vi "COMI DO Put One.vi"(9 "status":i32, 10 "ch":i32, 11 "hDevice":u32) -> (2 "function return":i32, 3 "hDevice out":u32)   [LabVIEW 2017, in "Comidll.lvlib"]
doc: "int (COMI_DO_PutOne) (HANDLE hDevice, int ch, int status);"
uses:
  <userlib>/Comidll/Comidll.lvlib
  <userlib>/Comidll/Comidll.dll
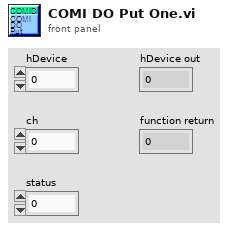
[diagram p1: front panel]
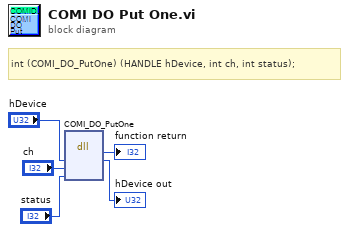
[diagram p0: block diagram]
diagram:
  # "int\t(COMI_DO_PutOne) (HANDLE hDevice, int ch, int status);"
  n1 = dll-call lib="C:/Program Files/National Instruments/LabVIEW 2017/user.lib/Comidll/Comidll.*" fn="COMI_DO_PutOne"("hDevice"="hDevice", "ch"="ch", "status"="status") -> (→"function return":i32, "hDevice"=→"hDevice out":u32)  [unwired: 5 in, 2 out]
